vi "Create.vi"(8 "error in (no error)":errorcluster, 9 "Dimension":refnum<class "Data.lvclass">, 10 "Raw":refnum<class "Data.lvclass">, 11 "Data":refnum<class "Data.lvclass">) -> (0 "error out":errorcluster, 3 "Signal out":refnum<class "Signal.lvclass">)   [LabVIEW 2012, in "MDSplus.lvlib" / "Signal.lvclass"]
uses:
  <vilib>/MDSplus/Classes/Data_Class/Compound_Class/Signal_Class/Signal.lvclass
  <vilib>/MDSplus/Classes/Data_Class/Data.lvclass
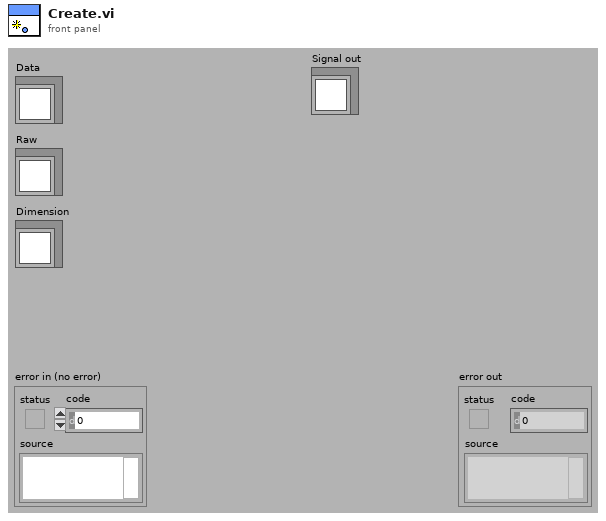
[diagram p1: front panel]
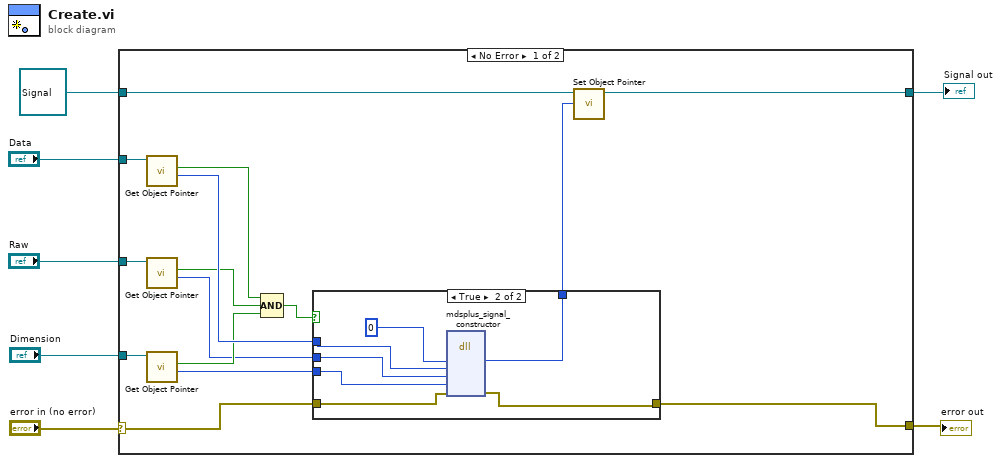
[diagram p0: block diagram]
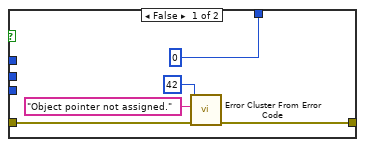
[diagram p2: hidden frame]
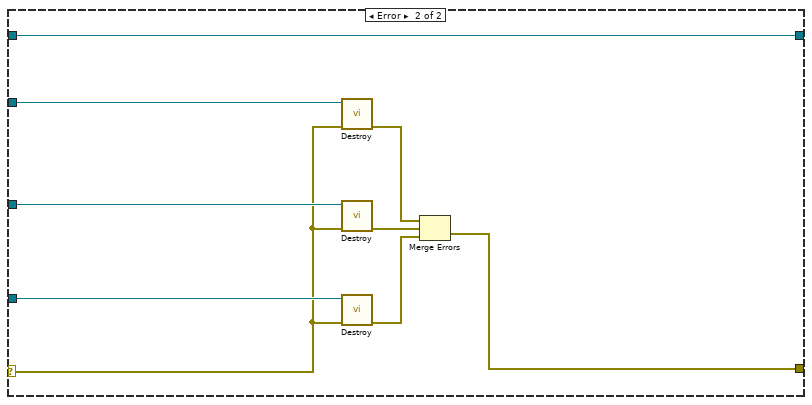
[diagram p3: hidden frame]
diagram:
  n1 = case shown="No Error" "error in (no error)" {
    selector: "error in (no error)" -> [w18 w36]
    tunnel: [w12 w43] -> w2
    tunnel: refnum<class "Signal.lvclass"> refnum ("Range in") -> [w13 w43]
    tunnel: "Data" -> [w22 w42]
    tunnel: "Raw" -> [w21 w41]
    tunnel: "Dimension" -> [w20 w40]
    tunnel: [w8 w35] -> w1
    frame No Error {
      n2 = call-dynamic "Get Object Pointer.vi"("Data in"=w22) -> ("Object Pointer"=w19:i64, "Assigned object pointer?"=w17:bool)  [unwired: 8 in, 1 out]
      n3 = call-dynamic "Get Object Pointer.vi"("Data in"=w21) -> ("Object Pointer"=w11:i64, "Assigned object pointer?"=w14:bool)  [unwired: 8 in, 1 out]
      n4 = call-dynamic "Get Object Pointer.vi"("Data in"=w20) -> ("Object Pointer"=w10:i64, "Assigned object pointer?"=w16:bool)  [unwired: 8 in, 1 out]
      n5 = Compound Arithmetic op=AND(w17, w14, w16) -> (w15:bool)
      n6 = case shown="True" w15 {
        tunnel: w19 -> [_ w29]
        tunnel: w18 -> [w25 w34]
        tunnel: [w24 w33] -> w8
        tunnel: w11 -> [_ w31]
        tunnel: w10 -> [_ w30]
        tunnel: [i64 0 ("lvRangePtr") w28] -> w9
        frame False {
          n7 = call <vilib>:"Error Cluster From Error Code.vi"("error in (no error)"=w25, "error message (\"\")"="Object pointer not assigned." ("error message (\"\")"), "error code (0)"=42) -> ("error out"=w24:errorcluster)  [unwired: 6 in]
        }
        frame True {
          n8 = dll-call lib="MDSobjectsLVShr" fn="mdsplus_signal_constructor"("lvSignalPtr"=i64 0 ("lvRangePtr"), "lvDataPtrIn"=w29, "lvRawPtrIn"=w31, "lvDimPtrIn"=w30, "error"=w34) -> ("lvSignalPtr"=w28:i64, "error"=w33:errorcluster)  [unwired: 7 in, 2 out]
        }
      }
      n9 = call-dynamic "Set Object Pointer.vi"("Object Pointer"=w9, "Data in"=w13) -> ("Data out"=w12:refnum<class "Signal.lvclass">)  [unwired: 9 in]
    }
    frame Error {
      n10 = call-dynamic "Destroy.vi"("error in (no error)"=w36, "Data in"=w42) -> ("error out"=w37:errorcluster)  [unwired: 9 in]
      n11 = call-dynamic "Destroy.vi"("error in (no error)"=w36, "Data in"=w41) -> ("error out"=w39:errorcluster)  [unwired: 9 in]
      n12 = call-dynamic "Destroy.vi"("error in (no error)"=w36, "Data in"=w40) -> ("error out"=w38:errorcluster)  [unwired: 9 in]
      n13 = Merge Errors(w37, w39, w38) -> (w35:errorcluster)
    }
  }
  "error out" <- w1
  "Signal out" <- w2
